vi "ReadChangedLVFilesList.vi"(8 "error in (no error)":errorcluster) -> (0 "error out":errorcluster, 3 "ChangedLVFilesList":path[](array[path]))   [LabVIEW 2019, in "DepsWatch.lvlib"]
uses:
  DepsWatch.lvlib
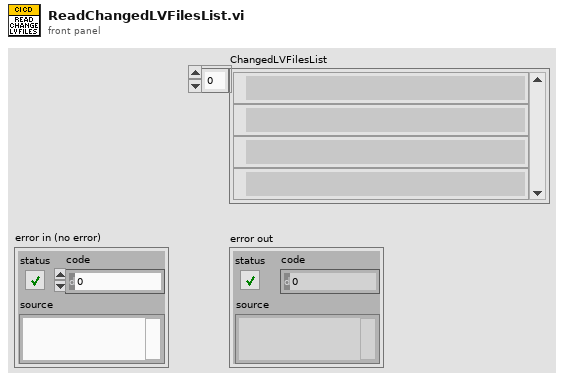
[diagram p1: front panel]
types:
  T1 = enum16{"open", "replace", "create", "open or create", "replace or create", "replace or create with confirmation"}
  T2 = typedef "DepsWatch.lvlib/CICDPathConfigs.ctl" = cluster{"GlobalIncludePaths":path[], "GlobalExcludePaths":path[], "BuildSpecsIncludePaths":path[], "ActualDepsIncludePaths":path[], "WorkspacePath":path, "SourceFolderPaths":path[], "ChangedFilesLogpaths":map{string, path}}
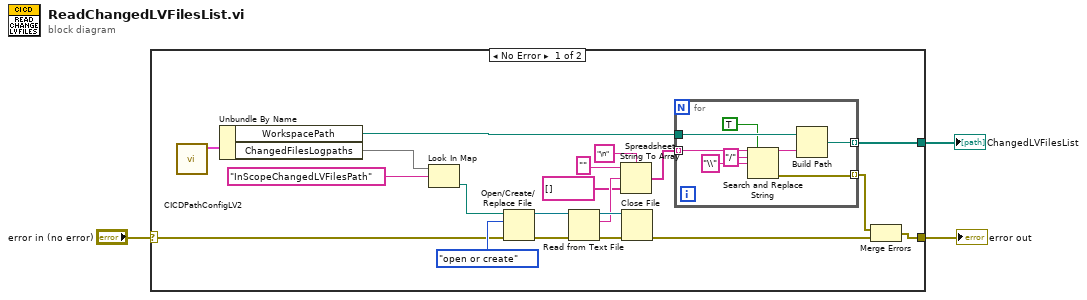
[diagram p0: block diagram]
diagram:
  n1 = case shown="No Error" "error in (no error)" {
    selector: "error in (no error)" -> [w14 w32]
    tunnel: [w5 w32] -> w2
    tunnel: [w6 _] -> w1
    frame No Error {
      n2 = call "CICDPathConfigLV2.vi"() -> ("CICD Path Config Out"=w23:T2)  [unwired: 11 in]
      n3 = Unbundle By Name(w23) -> ("WorkspacePath"=w8:path, "ChangedFilesLogpaths"=w21:map{string, path})
      n4 = Look In Map(map=w21, key="InScopeChangedLVFilesPath") -> (value=w13:path)  [unwired: 1 in, 1 out]
      n5 = Open/Create/Replace File(file path (use dialog)=w13, error in=w14, operation (0:open)=T1."open or create") -> (refnum out=w19:refnum<file>, error out=w18:errorcluster)  [unwired: 3 in, 1 out]
      n6 = Read from Text File(file (use dialog)=w19, error in=w18) -> (refnum out=w17:refnum<file>, text=w15:string, error out=w16:errorcluster)  [unwired: 2 in, 1 out]
      n7 = Spreadsheet String To Array(delimiter (Tab)="\n", format string="", spreadsheet string=w15, array type (2D Dbl)=string[] []) -> (array=w7:string[])
      n8 = Close File(refnum=w17, error in=w16) -> (error out=w9:errorcluster)  [unwired: 1 out]
      n9 = for {
        tunnel: w8 -> [w31]
        tunnel: w7 -> [w29] mode=indexing
        tunnel: [w30] -> w6 mode=indexing
        tunnel: [w25] -> w4 mode=indexing
        n10 = Search and Replace String(replace all?=TRUE ("replace all? (F)"), input string=w29, search string="/", replace string="\\" ("replace string (\"\")")) -> (result string=w26:string, error out=w25:errorcluster)  [unwired: 4 in, 2 out]
        n11 = Build Path(base path=w31, name or relative path=w26) -> (appended path=w30:path)
      }
      n12 = Merge Errors(w4, w9) -> (w5:errorcluster)
    }
    frame Error {
    }
  }
  "ChangedLVFilesList" <- w1
  "error out" <- w2
